vi "报警XML解析.vi"(8 "error in (no error)":errorcluster caption="错误输入（无错误）", 11 "筛选输入":T2={"componentParentName"="斯坦道营养盐", "componentName"="", "equipVersion"="B", "Code"=""}) -> (0 "error out":errorcluster caption="错误输出", 3 "alarm":T1)   [LabVIEW 2016, in "Alarm interface.lvlib"]
uses:
  Alarm interface.lvlib
  <vilib>/xml/Load XML File.vi
  <vilib>/xml/Close Reference(Node).vi
  <vilib>/xml/NI_XML.lvlib
  <resource>/objmgr/DOMUserDefRef.rc
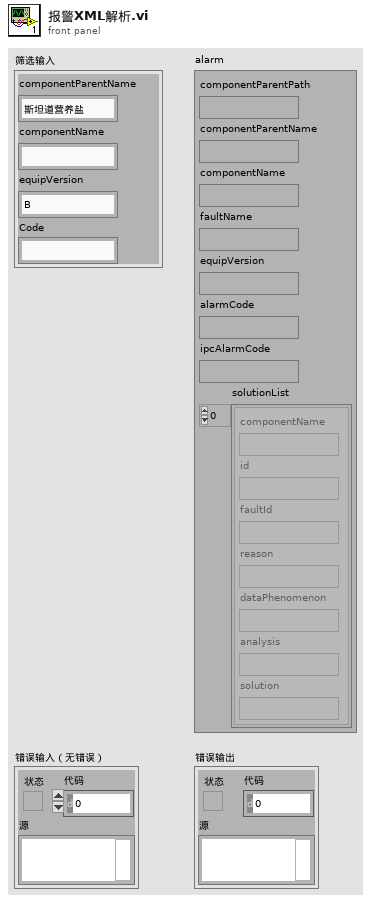
[diagram p1: front panel]
types:
  T1 = cluster{"componentParentPath":string, "componentParentName":string, "componentName":string, "faultName":string, "equipVersion":string, "alarmCode":string, "ipcAlarmCode":string, "solutionList":cluster{"componentName":string, "id":string, "faultId":string, "reason":string, "dataPhenomenon":string, "analysis":string, "solution":string}[]}
  T2 = cluster{"componentParentName":string, "componentName":string, "equipVersion":string, "Code":string}
  T3 = cluster{"node text":string, "node text":string, "node text":string, "node text":string, "node text":string, "node text":string, "node text":string}
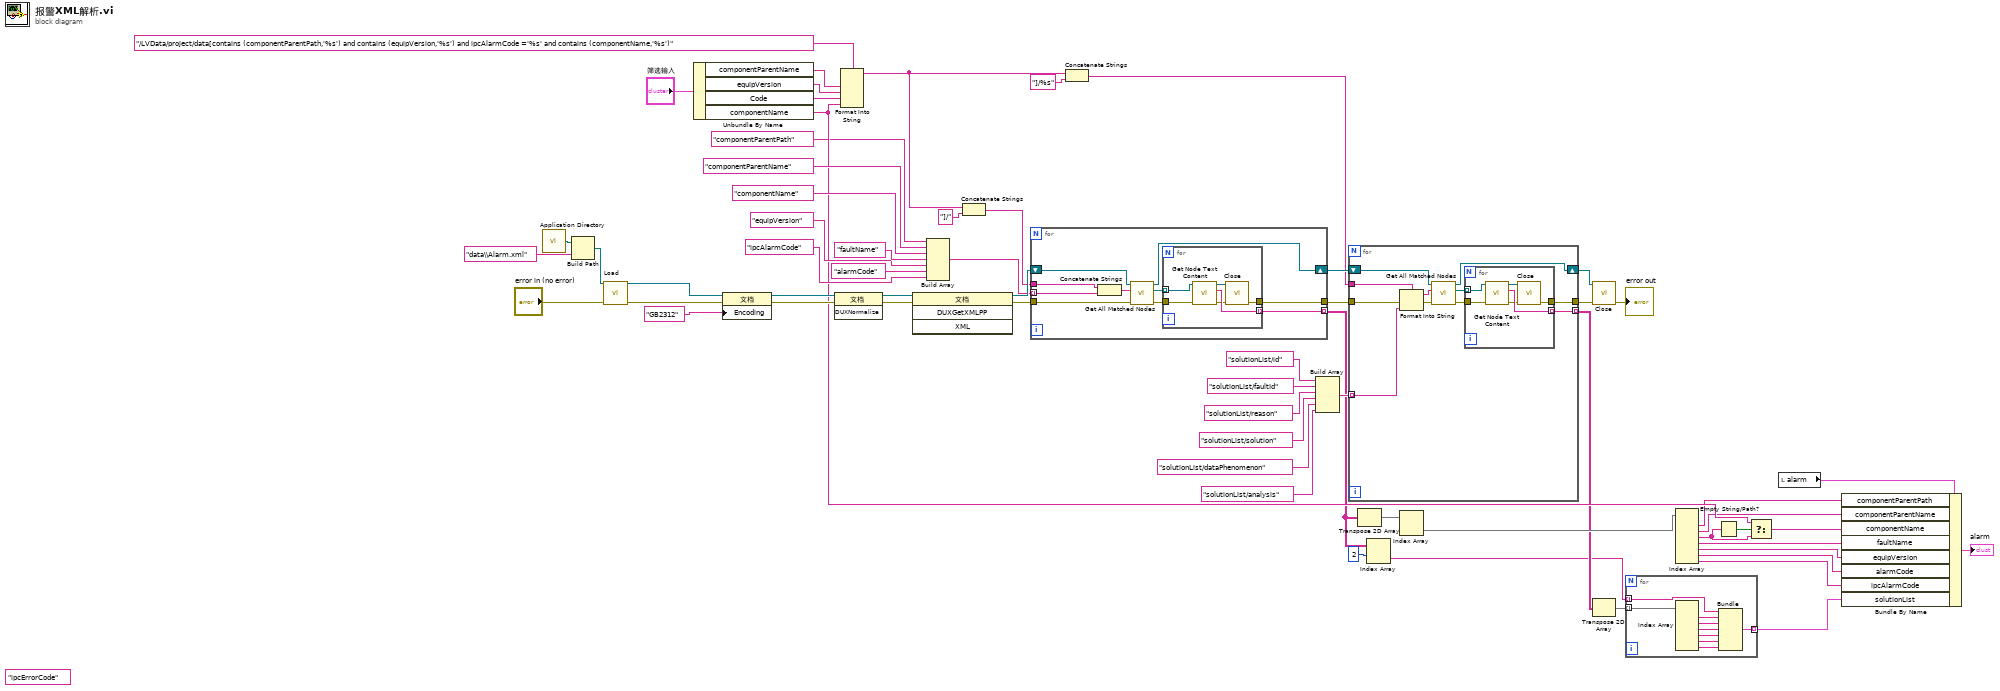
[diagram p0: block diagram]
diagram:
  (unwired) "ipcErrorCode"
  n1 = call <vilib>:"Application Directory.vi"() -> ("Application Directory"=w34:path)
  n2 = Build Path(base path=w34, name or relative path="data\\Alarm.xml" ("字符串")) -> (appended path=w32:path)
  n3 = call-poly <vilib>:"Load.vi"("path to XML document"=w32, "error in (no error)"="error in (no error)") -> ("DOM document out"=w60:refnum<k20>, "error out"=w59:errorcluster)  [unwired: 11 in, 1 out]
  n4 = Unbundle By Name("筛选输入") -> ("componentParentName"=w35:string, "equipVersion"=w29:string, "Code"=w30:string, "componentName"=w27:string)
  n5 = property on="属性节点" class="文档"(reference=w60, error in=w59, "Encoding"="GB2312" ("文档编码")) -> (reference out=w62:refnum<k20>, error out=w61:errorcluster)
  n6 = invoke on="调用节点" class="文档" method="DUXNormalize"(reference=w62, error in=w61) -> (reference out=w58:refnum<k20>, error out=w57:errorcluster)  [unwired: 1 in, 1 out]
  n7 = Format Into String(format string="/LVData/project/data[contains (componentParentPath,'%s') and contains (equipVersion,'%s') and ipcAlarmCode ='%s' and contains (componentName,'%s')" ("字符串"), w35, w29, w30, w27) -> (resulting string=w31:string)  [unwired: 2 in, 1 out]
  n8 = invoke on="调用节点" class="文档" method="DUXGetXMLPP"(reference=w58, error in=w57) -> (reference out=w50:refnum<k20>, error out=w39:errorcluster)  [unwired: 2 in, 2 out]
  n9 = Build Array("componentParentPath", "componentParentName", "componentName", "faultName", "equipVersion", "alarmCode", "ipcAlarmCode") -> (w49:string[])
  n10 = Concatenate Strings(w31, "]/" ("字符串")) -> (w44:string)
  n11 = for {
    tunnel: w44 -> [w67]
    tunnel: w49 -> [w66] mode=indexing
    tunnel: [w71] -> w1 mode=indexing
    tunnel: [w68] -> w40
    tunnel: w39 -> [w65]
    shift-right: [w70] -> w48
    shift-left: w50 -> [w73]
    n12 = Concatenate Strings(w67, w66) -> (w64:string)
    n13 = call <vilib>:"Get All Matched Nodes.vi"("error in (no error)"=w65, "XPath expression"=w64, "node in"=w73) -> ("error out"=w69:errorcluster, "node result array"=w72:refnum<k20>[], "node out"=w70:refnum<k20>)  [unwired: 6 in]
    n14 = for {
      tunnel: w72 -> [w79] mode=indexing
      tunnel: [w78] -> w71 mode=indexing
      tunnel: w69 -> [w77]
      tunnel: [w74] -> w68
      n15 = call <vilib>:"Get Node Text Content.vi"("error in (no error)"=w77, "node in"=w79) -> ("error out"=w75:errorcluster, "node text"=w78:string, "node out"=w76:refnum<k20>)  [unwired: 7 in]
      n16 = call-poly <vilib>:"Close.vi"("error in (no error)"=w75, "node"=w76) -> ("error out"=w74:errorcluster)  [unwired: 7 out]
    }
  }
  n17 = Concatenate Strings(w31, "]/%s" ("字符串")) -> (w42:string)
  n18 = Build Array("solutionList/id" ("XPath expression"), "solutionList/faultId" ("XPath expression"), "solutionList/reason" ("XPath expression"), "solutionList/solution" ("XPath expression"), "solutionList/dataPhenomenon" ("XPath expression"), "solutionList/analysis" ("XPath expression")) -> (w9:string[])
  n19 = for {
    tunnel: w42 -> [w90]
    tunnel: w9 -> [w89] mode=indexing
    tunnel: [w85] -> w8 mode=indexing
    tunnel: w40 -> [w83]
    tunnel: [w80] -> w38
    shift-right: [w84] -> w47
    shift-left: w48 -> [w87]
    n20 = Format Into String(format string=w90, error in=w83, w89) -> (resulting string=w86:string, error out=w82:errorcluster)  [unwired: 1 in]
    n21 = call <vilib>:"Get All Matched Nodes.vi"("error in (no error)"=w82, "XPath expression"=w86, "node in"=w87) -> ("error out"=w81:errorcluster, "node result array"=w88:refnum<k20>[], "node out"=w84:refnum<k20>)  [unwired: 6 in]
    n22 = for {
      tunnel: w88 -> [w96] mode=indexing
      tunnel: [w95] -> w85 mode=indexing
      tunnel: w81 -> [w94]
      tunnel: [w91] -> w80
      n23 = call <vilib>:"Get Node Text Content.vi"("error in (no error)"=w94, "node in"=w96) -> ("error out"=w92:errorcluster, "node text"=w95:string, "node out"=w93:refnum<k20>)  [unwired: 7 in]
      n24 = call-poly <vilib>:"Close.vi"("error in (no error)"=w92, "node"=w93) -> ("error out"=w91:errorcluster)  [unwired: 7 out]
    }
  }
  n25 = Transpose 2D Array(2D array=w1) -> (transposed array=w46:string[][])
  n26 = Index Array(array=w1, index (row)=2 ("索引")) -> (element=w4:string[])  [unwired: 1 in]
  n27 = Index Array(array=w46) -> (element=w26:string[])  [unwired: 2 in]
  n28 = call-poly <vilib>:"Close.vi"("error in (no error)"=w38, "node"=w47) -> ("error out"=→"error out":errorcluster)  [unwired: 7 out]
  n29 = Transpose 2D Array(2D array=w8) -> (transposed array=w7:string[][])
  n30 = for {
    tunnel: w7 -> [w105] mode=indexing
    tunnel: [w100] -> w2 mode=indexing
    tunnel: w4 -> [w97] mode=indexing
    n31 = Index Array(array=w105) -> (element #1=w104:string, element #2=w103:string, element #3=w102:string, element #4=w101:string, element #5=w99:string, element #6=w98:string)  [unwired: 6 in]
    n32 = Bundle("node text"=w97, "node text"=w104, "node text"=w103, "node text"=w102, "node text"=w101, "node text"=w99, "node text"=w98) -> (w100:T3)  [unwired: 1 in]
  }
  n33 = Index Array(array=w26) -> (element #1=w14:string, element #2=w25:string, element #3=w18:string, element #4=w16:string, element #5=w24:string, element #6=w23:string, element #7=w22:string)  [unwired: 7 in]
  n34 = Empty String/Path?(string/path=w18) -> (empty?=w21:bool)
  n35 = Select(t=w27, s=w21, f=w18) -> (s? t:f=w17:string)
  n36 = local read "alarm"() -> (w19:T1)
  n37 = Bundle By Name(cluster=w19, "componentParentPath"=w14, "componentParentName"=w25, "componentName"=w17, "faultName"=w16, "equipVersion"=w24, "alarmCode"=w23, "ipcAlarmCode"=w22, "solutionList"=w2) -> (→"alarm":T1)
